vi "change_color_palette.vi"(8 "error in (no error)":errorcluster, 10 "raw channel index":i32, 11 "DisplayDL090216 in":refnum<class "DisplayDL090216.lvclass">) -> (0 "error out":errorcluster, 3 "DisplayDL090216 out":refnum<class "DisplayDL090216.lvclass">)   [LabVIEW 2010, in "DisplayDL090216.lvclass"]
uses:
  DisplayDL090216.lvclass
  common/classes/ColorOverlay/ColorOverlay/ColorOverlay.lvclass
  common/classes/Image/Image/Image.lvclass
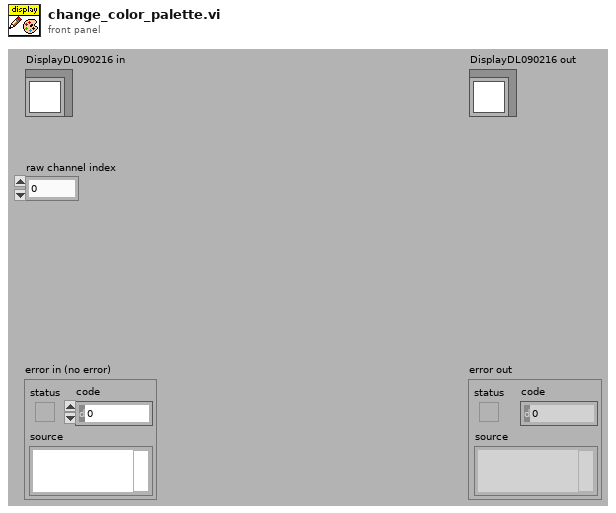
[diagram p1: front panel]
types:
  T1 = typedef "IMAQ Image.ctl" = refnum<image>
  T2 = cluster{"Numeric":u32, "Numeric":u32, "Numeric":u32}[]
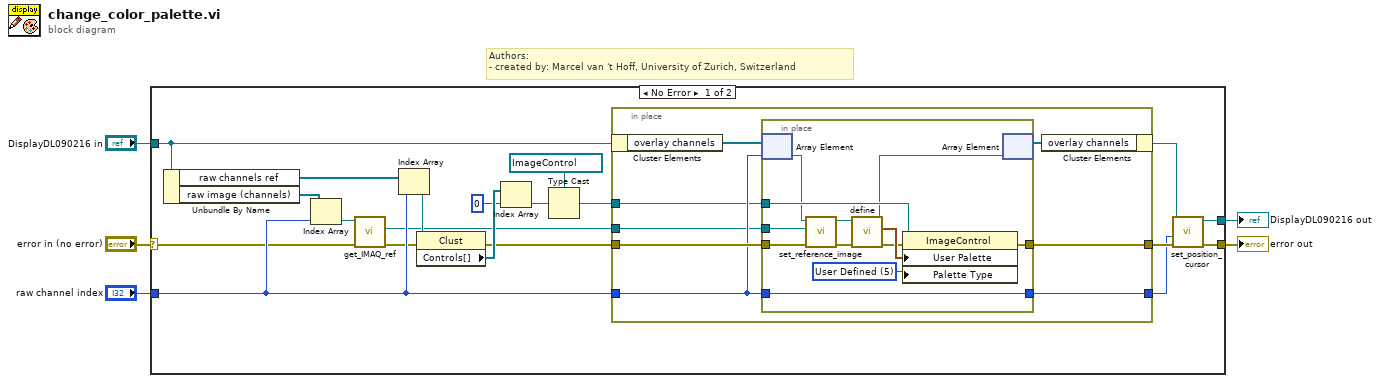
[diagram p0: block diagram]
diagram:
  # "Authors: \n- created by: Marcel van 't Hoff, University of Zurich, Switzerland"
  n1 = case shown="No Error" "error in (no error)" {
    selector: "error in (no error)" -> [w6 w47]
    tunnel: [w16 w47] -> w4
    tunnel: [w17 w46] -> w2
    tunnel: "DisplayDL090216 in" -> [w20 w46]
    tunnel: "raw channel index" -> [w11 _]
    frame No Error {
      n2 = Unbundle By Name(w20) -> ("raw channels ref"=w22:refnum<vi>[], "raw image (channels)"=w12:refnum<class "Image.lvclass">[])
      n3 = Index Array(array=w12, index=w11) -> (element=w10:refnum<class "Image.lvclass">)
      n4 = call-dynamic "get_IMAQ_ref.vi"("error in (no error)"=w6, "Image.lvclass in"=w10) -> ("error out"=w8:errorcluster, "Image"=w9:T1)  [unwired: 8 out]
      n5 = Index Array(array=w22, index=w11) -> (element=w21:refnum<vi>)
      n6 = property class="Clust"(reference=w21, error in=w8) -> (error out=w7:errorcluster, "Controls[]"=w25:refnum<vi>[])  [unwired: 1 out]
      n7 = Index Array(array=w25, index=0) -> (element=w24:refnum<vi>)
      n8 = Type Cast(type=refnum<vi> refnum ("histogram out"), x=w24) -> (*(type *) &x=w19:refnum<vi>)
      n9 = in-place {
        in-place-border: w11 -> [w28]
        in-place-border: [w30] -> w15
        in-place-border: w19 -> [w27]
        in-place-border: w7 -> [w31]
        in-place-border: [w29] -> w14
        in-place-border: w9 -> [w26]
        n10 = in-place-cluster #1(w20) -> ("overlay channels"=w33:refnum<class "ColorOverlay.lvclass">[])
        n11 = in-place {
          in-place-border: w27 -> [w42]
          in-place-border: w31 -> [w36]
          in-place-border: [w40] -> w30
          in-place-border: [w39] -> w29
          in-place-border: w28 -> [w39]
          in-place-border: w26 -> [w34]
          w44 = u32 5 items=["Grayscale", "Binary", "Gradient", "Rainbow", "Temperature", "User Defined"] ("Palette:Palette Type")
          n12 = in-place-array #2(w33, w28) -> (w38:refnum<class "ColorOverlay.lvclass">)
          n13 = call-dynamic "set_reference_image.vi"("error in (no error)"=w36, "reference image"=w34, "ColorOverlay in"=w38) -> ("error out"=w35:errorcluster, "ColorOverlay out"=w37:refnum<class "ColorOverlay.lvclass">)  [unwired: 7 in]
          n14 = call-dynamic "define.vi"("error in (no error)"=w35, "ColorOverlay in"=w37) -> ("error out"=w43:errorcluster, "color cluster out"=w45:T2, "ColorOverlay out"=w41:refnum<class "ColorOverlay.lvclass">)  [unwired: 7 in]
          n15 = property class="ImageControl"(reference=w42, error in=w43, "User Palette"=w45, "Palette Type"=w44) -> (error out=w40:errorcluster)  [unwired: 1 out]
          n16 = in-place-array #2(w41) -> (w32:refnum<class "ColorOverlay.lvclass">[])  [unwired: 1 out]
        }
        n17 = in-place-cluster #1("overlay channels"=w32) -> (w18:refnum<class "DisplayDL090216.lvclass">)
      }
      n18 = call-dynamic "set_position_cursor.vi"("error in (no error)"=w15, "raw channel index"=w14, "DisplayDL090216 in"=w18) -> ("error out"=w16:errorcluster, "DisplayDL090216 out"=w17:refnum<class "DisplayDL090216.lvclass">)  [unwired: 7 in]
    }
    frame Error {
    }
  }
  "error out" <- w4
  "DisplayDL090216 out" <- w2
